vi "L19.vi"() -> ()   [LabVIEW 2012]
uses:
  <vilib>/Utility/miscctls.llb/LVDateTimeRec.ctl
panel:
  out "number of replacements":i32
  in  "date time rec":T1={"fractional second"=1.0, "second"=1, "minute"=1, "hour"=1, "day of month"=1, "month"=1, "year"=2000, "day of week"=0, "day of year"=0, "DST"=0}
  out "time stamp":timestamp
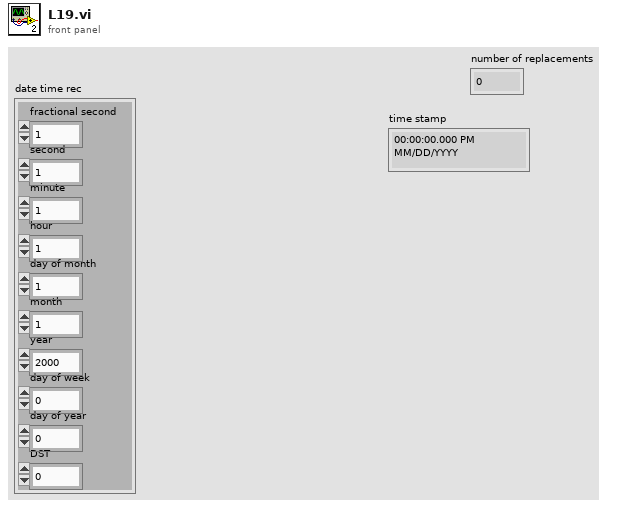
[diagram p1: front panel]
types:
  T1 = typedef "LVDateTimeRec.ctl" = cluster{"fractional second":dbl, "second":i32, "minute":i32, "hour":i32, "day of month":i32, "month":i32, "year":i32, "day of week":i32, "day of year":i32, "DST":i32}
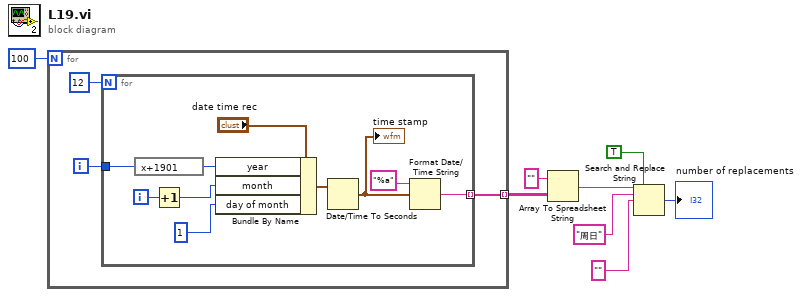
[diagram p0: block diagram]
diagram:
  n1 = for {
    N: 100 -> [_]
    tunnel: [w9] -> w7 mode=indexing
    i -> [w11]
    n2 = for {
      N: 12 -> [_]
      tunnel: w11 -> [w14]
      tunnel: [w13] -> w9 mode=indexing
      i -> [w16]
      n3 = expression code="x+1901"(w14) -> (w12:i32)
      n4 = Increment(x=w16) -> (x+1=w15:i32)
      n5 = Bundle By Name(cluster="date time rec", "year"=w12, "month"=w15, "day of month"=1) -> (w17:T1)
      n6 = Date/Time To Seconds(2:w17) -> (0:w20:timestamp)  [unwired: 1 in]
      "time stamp" <- w20
      n7 = Format Date/Time String(time format string (%c)="%a", seconds (now)=w20) -> (date/time string=w13:string)  [unwired: 1 in]
    }
  }
  n8 = Array To Spreadsheet String(array=w7, 3:"" ("format string")) -> (spreadsheet string=w5:string)  [unwired: 1 in]
  n9 = Search and Replace String(replace all?=TRUE ("replace all? (F)"), input string=w5, search string="周日", replace string="" ("replace string (\"\")")) -> (number of replacements=→"number of replacements":i32)  [unwired: 4 in, 3 out]
